vi "WLAN - niVST - RFSA - Gain and Trigger Settings.vi"(0 "instrument handle":refnum<k15>, 7 "External Attenuation (dB)":dbl, 11 "error in":errorcluster, 12 "NI HW":bool=TRUE) -> (4 "instrument handle":refnum<k15>, 15 "error out":errorcluster)   [LabVIEW 2011]
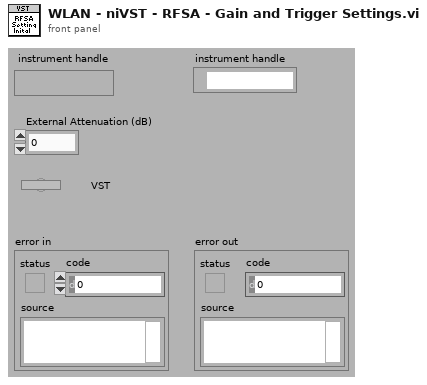
[diagram p1: front panel]
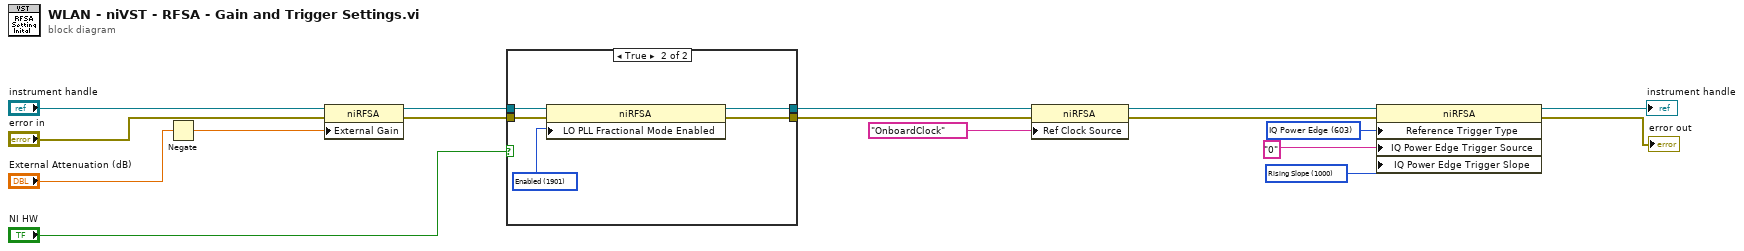
[diagram p0: block diagram]
diagram:
  w10 = 1000 items=["Rising Slope"=1000, "Falling Slope"=1001] ("Triggers:Ref:IQ Power Edge:Slope")
  w12 = 603 items=["None"=600, "Digital Edge"=601, "IQ Power Edge"=603, "Software"=604, "IQ Analog Edge"=605] ("Triggers:Ref:Type")
  n1 = Negate(x="External Attenuation (dB)") -> (-x=w14:dbl)
  n2 = property on="Property Node" class="niRFSA"(reference="instrument handle", error in="error in", "External Gain"=w14) -> (reference out=w5:refnum<k15>, error out=w2:errorcluster)
  n3 = case shown="True" "NI HW" {
    tunnel: w5 -> [w19 w24]
    tunnel: [w19 w23] -> w4
    tunnel: [w18 w22] -> w3
    tunnel: w2 -> [w18 w21]
    frame False {
    }
    frame True {
      w20 = 1901 items=["Disabled"=1900, "Enabled"=1901] ("RF-RIO:Signal Path:LO PLL Fractional Mode Enabled")
      n4 = property on="Property Node" class="niRFSA"(reference=w24, error in=w21, "LO PLL Fractional Mode Enabled"=w20) -> (reference out=w23:refnum<k15>, error out=w22:errorcluster)
    }
  }
  n5 = property class="niRFSA"(reference=w4, error in=w3, "Ref Clock Source"="OnboardClock" ("Clocking:Ref Clock Source")) -> (reference out=w9:refnum<k15>, error out=w8:errorcluster)
  n6 = property class="niRFSA"(reference=w9, error in=w8, "Reference Trigger Type"=w12, "IQ Power Edge Trigger Source"="0" ("source"), "IQ Power Edge Trigger Slope"=w10) -> (reference out=→"instrument handle":refnum<k15>, error out=→"error out":errorcluster)
